vi "RCMDatumToMenuItems.vi"(8 "error in (no error)":errorcluster, 11 "rcm datum":T1[](array[typedef])) -> (0 "error out":errorcluster, 3 "menu items":refnum<class "menu item.lvclass">[](array[class]))   [LabVIEW 2009]
uses:
  Type Definitions/RCMData.ctl
  Class/Menu Item/menu item.lvclass
  Class/Text Item/text item.lvclass
  Class/Separator Item/separator item.lvclass
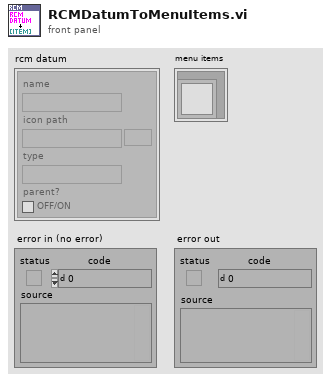
[diagram p1: front panel]
types:
  T1 = typedef "RCMData.ctl" = cluster{"name":string, "icon path":path, "type":string, "parent?":bool}
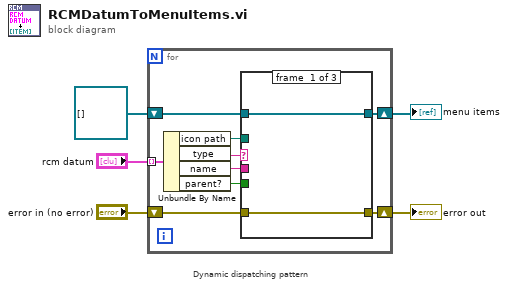
[diagram p0: block diagram]
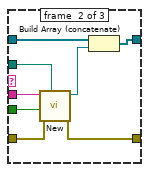
[diagram p2: hidden frame]
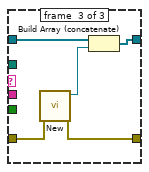
[diagram p3: hidden frame]
diagram:
  # "Dynamic dispatching pattern"
  n1 = for {
    tunnel: "rcm datum" -> [w14] mode=indexing
    shift-right: [w11] -> w2
    shift-left: refnum<class "menu item.lvclass">[] [] ("menu items") -> [w12]
    shift-right: [w6] -> w1
    shift-left: "error in (no error)" -> [w7]
    n2 = Unbundle By Name(w14) -> ("icon path"=w9:path, "type"=w13:string, "name"=w10:string, "parent?"=w8:bool)
    n3 = case shown="\"Separator\"" w13 {
      tunnel: w12 -> [w16 w24 w29]
      tunnel: [w16 w23 w28] -> w11
      tunnel: w10 -> [_ w21 _]
      tunnel: w9 -> [_ w20 _]
      tunnel: w8 -> [_ w19 _]
      tunnel: w7 -> [w15 w18 w26]
      tunnel: [w15 w17 w25] -> w6
      frame #0 {
      }
      frame #1 {
        n4 = call "New.vi"("parent"=w19, "icon path"=w20, "error in (no error)"=w18, "item name"=w21) -> ("error out"=w17:errorcluster, "text item out"=w22:refnum<class "text item.lvclass">)  [unwired: 6 in]
        n5 = Build Array (concatenate)(w24, w22) -> (w23:refnum<class "menu item.lvclass">[])
      }
      frame #2 {
        n6 = call "New.vi"("error in (no error)"=w26) -> ("error out"=w25:errorcluster, "separator item out"=w27:refnum<class "separator item.lvclass">)  [unwired: 9 in]
        n7 = Build Array (concatenate)(w29, w27) -> (w28:refnum<class "menu item.lvclass">[])
      }
    }
  }
  "menu items" <- w2
  "error out" <- w1
